vi "parse_quaternion_roslv.vi"(4 "error in":errorcluster, 7 "msg in":string) -> (0 "error out":errorcluster, 2 "Quaternion":cluster{"x":dbl, "y":dbl, "z":dbl, "w":dbl}, 3 "msg out":string)   [LabVIEW 2014]
doc: "Parses a message into a quaternion"
uses:
  std_msgs/subs/parse_float64_scalar_roslv.vi
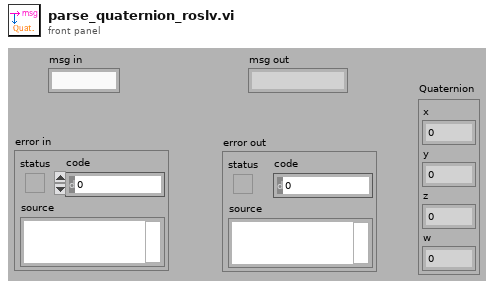
[diagram p1: front panel]
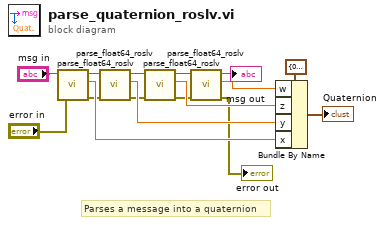
[diagram p0: block diagram]
diagram:
  # "Parses a message into a quaternion"
  n1 = call-poly "parse_float64_roslv.vi"("error in"="error in", "msg in"="msg in") -> ("error out"=w4:errorcluster, "number"=w8:dbl, "msg out"=w14:string)  [unwired: 3 in]
  n2 = call-poly "parse_float64_roslv.vi"("error in"=w4, "msg in"=w14) -> ("error out"=w3:errorcluster, "number"=w9:dbl, "msg out"=w12:string)  [unwired: 3 in]
  n3 = call-poly "parse_float64_roslv.vi"("error in"=w3, "msg in"=w12) -> ("error out"=w2:errorcluster, "number"=w10:dbl, "msg out"=w13:string)  [unwired: 3 in]
  n4 = call-poly "parse_float64_roslv.vi"("error in"=w2, "msg in"=w13) -> ("error out"=→"error out":errorcluster, "number"=w11:dbl, "msg out"=→"msg out":string)  [unwired: 3 in]
  n5 = Bundle By Name(cluster=cluster{"x":dbl, "y":dbl, "z":dbl, "w":dbl} {"x"=0.0, "y"=0.0, "z"=0.0, "w"=0.0} ("Quaternion"), "w"=w11, "z"=w10, "y"=w9, "x"=w8) -> (→"Quaternion":cluster{"x":dbl, "y":dbl, "z":dbl, "w":dbl})
